vi "Create Message.vi"(7 "Action":T1=enum."Scan Disable", 8 "error in (no error)":errorcluster, 11 "Telnet V2 in":refnum<class "Telnet V2.lvclass">) -> (0 "error out":errorcluster, 2 "Message Out":string)   [LabVIEW 2018, in "Telnet V2.lvlib" / "Telnet V2.lvclass"]
uses:
  Telnet V2.lvclass
  C:/AME Test Engineering/LabVIEW/PPLs/LiDAR/Parent/LiDAR.lvlibp/LiDAR.lvclass
  Controls/enum_Telnet_Actions.ctl
  PPLs/Configuration/Configuration.lvlibp/Configuration.lvclass
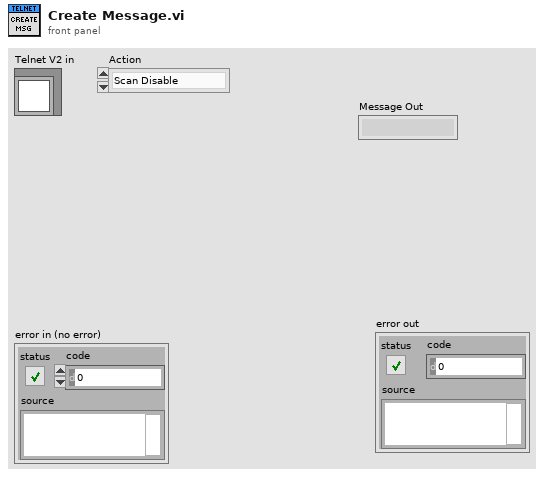
[diagram p1: front panel]
types:
  T1 = typedef "Telnet V2.lvlib/Telnet V2.lvclass/enum_Telnet_Actions.ctl" = enum16{"Scan Enable", "Scan Disable", "Active", "Standby", "Change EL Scan", "Change AZ Scan", "Set Data Algo", "Access System", "Access Laser", "Exit"}
  T2 = cluster{"Configuration":refnum<class "Configuration.lvclass">, "Azimuth":cluster{"Min >=-60":dbl, "Max <=+60 ":dbl}, "Elevation":cluster{"FOV":dbl, "Offset":dbl, "Scan Pattern":enum16{"Triangle", "Snap"}, "Frequency":dbl}, "Data Output":enum16{"Resim", "Point Cloud"}}
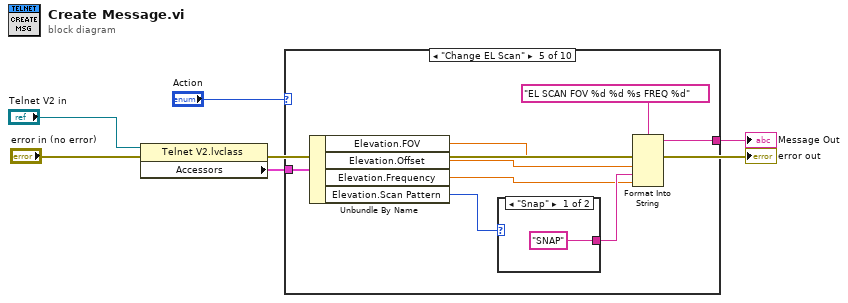
[diagram p0: block diagram]
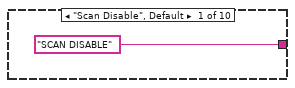
[diagram p2: hidden frame]
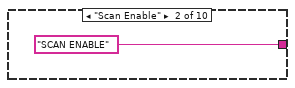
[diagram p3: hidden frame]
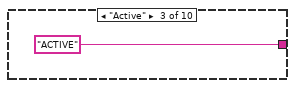
[diagram p4: hidden frame]
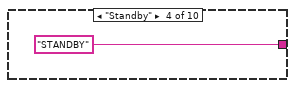
[diagram p5: hidden frame]
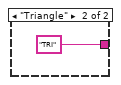
[diagram p6: hidden frame]
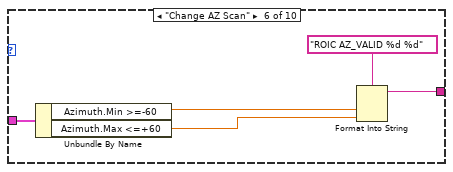
[diagram p7: hidden frame]
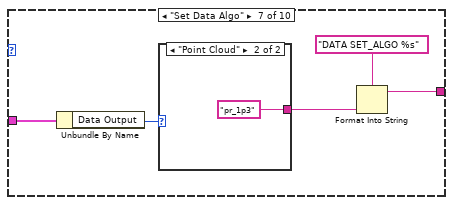
[diagram p8: hidden frame]
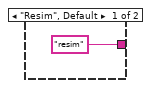
[diagram p9: hidden frame]
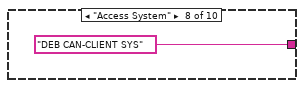
[diagram p10: hidden frame]
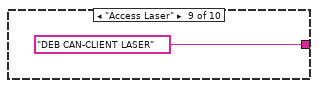
[diagram p11: hidden frame]
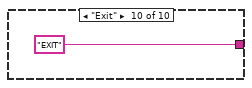
[diagram p12: hidden frame]
diagram:
  n1 = property class="Telnet V2.lvclass"(reference="Telnet V2 in", error in="error in (no error)") -> (error out=→"error out":errorcluster, "Accessors"=w6:T2)  [unwired: 1 out]
  n2 = case shown="\"Change EL Scan\"" "Action" {
    tunnel: w6 -> [_ _ _ _ w16 w23 w28 _ _ _]
    tunnel: ["SCAN DISABLE" "SCAN ENABLE" "ACTIVE" "STANDBY" w18 w25 w30 "DEB CAN-CLIENT SYS" "DEB CAN-CLIENT LASER" "EXIT"] -> w1
    frame "Scan Disable", Default {
    }
    frame "Scan Enable" {
    }
    frame "Active" {
    }
    frame "Standby" {
    }
    frame "Change EL Scan" {
      n3 = Unbundle By Name(w16) -> ("Elevation.FOV"=w15:dbl, "Elevation.Offset"=w14:dbl, "Elevation.Frequency"=w11:dbl, "Elevation.Scan Pattern"=w12:enum16{"Triangle", "Snap"})
      n4 = case shown="\"Snap\"" w12 {
        tunnel: ["SNAP" "TRI"] -> w13
        frame "Snap" {
        }
        frame "Triangle" {
        }
      }
      n5 = Format Into String(format string="EL SCAN FOV %d %d %s FREQ %d", w15, w14, w13, w11) -> (resulting string=w18:string)  [unwired: 2 in, 1 out]
    }
    frame "Change AZ Scan" {
      n6 = Unbundle By Name(w23) -> ("Azimuth.Min >=-60"=w22:dbl, "Azimuth.Max <=+60"=w21:dbl)
      n7 = Format Into String(format string="ROIC AZ_VALID %d %d", w22, w21) -> (resulting string=w25:string)  [unwired: 2 in, 1 out]
    }
    frame "Set Data Algo" {
      n8 = Unbundle By Name(w28) -> ("Data Output"=w27:enum16{"Resim", "Point Cloud"})
      n9 = case shown="\"Point Cloud\"" w27 {
        tunnel: ["resim" "pr_1p3"] -> w26
        frame "Resim", Default {
        }
        frame "Point Cloud" {
        }
      }
      n10 = Format Into String(format string="DATA SET_ALGO %s", w26) -> (resulting string=w30:string)  [unwired: 2 in, 1 out]
    }
    frame "Access System" {
    }
    frame "Access Laser" {
    }
    frame "Exit" {
    }
  }
  "Message Out" <- w1
